vi "ValveValues.vi"() -> ()   [LabVIEW 2013]
panel:
  in  "ValvesValues":bool[](array[boolean])
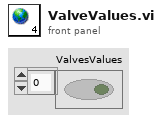
[diagram p1: front panel]
diagram:
